vi "Get Plugin Configuration.vi"(8 "error in (no error)":errorcluster, 11 "Component Configuration in":refnum<class "RDMA Configurations.lvclass">) -> (0 "error out":errorcluster, 2 "Plugin Configuration":refnum<class "Configuration.lvclass">, 3 "Component Configuration out":refnum<class "RDMA Configurations.lvclass">)   [LabVIEW 2020, in "RDMA.lvlib" / "RDMA Configurations.lvclass"]
uses:
  RDMA Configurations.lvclass
  DSF Core.lvlibp/Classes/Configuration/Configuration.lvclass
  Plugin/RDMA Plugin Configuration.lvclass
  C:/git/fmussi-niveristand-data-sharing-framework-custom-device-plugins/Components/DSF Core.lvlibp/Classes/Configuration/Configuration.lvclass
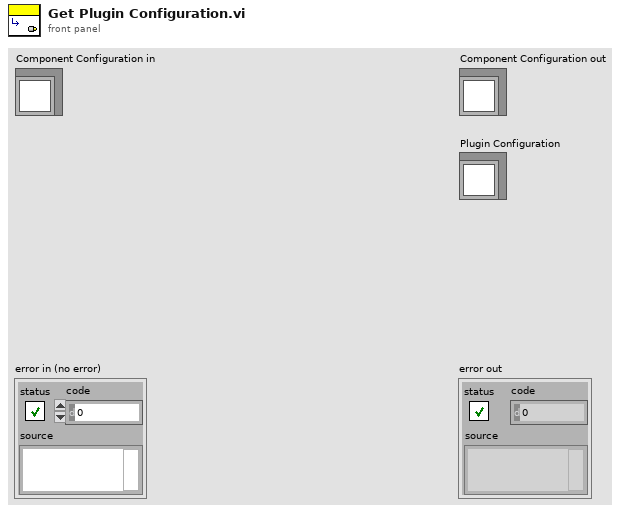
[diagram p1: front panel]
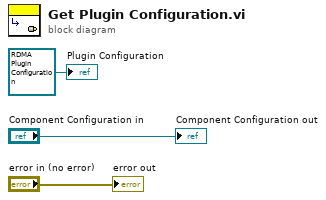
[diagram p0: block diagram]
diagram:
  "error out" <- "error in (no error)"
  "Component Configuration out" <- "Component Configuration in"
  "Plugin Configuration" <- refnum<class "RDMA Plugin Configuration.lvclass"> refnum ("RDMA.lvlib:RDMA Plugin Configuration.lvclass")
